vi "4.vi"() -> ()   [LabVIEW 2026]
uses:
  3global.vi
panel:
  out "Waveform Graph":dbl[][](graph)
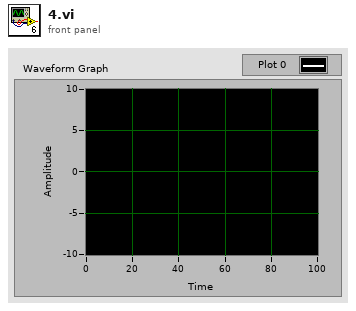
[diagram p1: front panel]
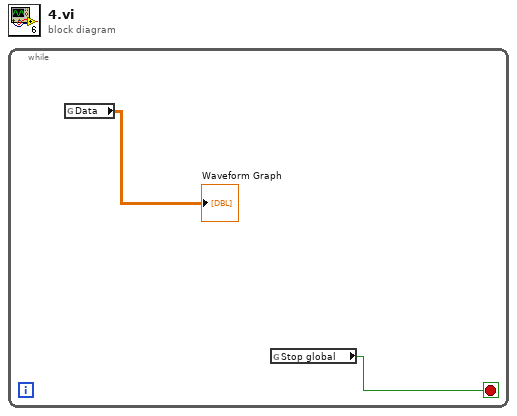
[diagram p0: block diagram]
diagram:
  n1 = while {
    stop <- w2 stop-if-true
    n2 = global read "3global.vi" "Data"() -> (→"Waveform Graph":dbl[][])
    n3 = global read "3global.vi" "Stop global"() -> (w2:bool)
  }
